vi "sorted data from csv.vi"(0 "cases CSV":string[][](array[string]), 2 "filter out":i32[](array[numeric]), 5 "US data":T1, 7 "Populations":i64[](array[numeric]), 9 "deaths CSV":string[][](array[string]), 11 "top selection":i32=5, 12 "SA data":T1, 13 "period in days to check":i32=7) -> (4 "ranked results":T2)   [LabVIEW 2019]
uses:
  <vilib>/Analysis/NI_AALPro.lvlib
panel:
  in  "last x days":i32=3
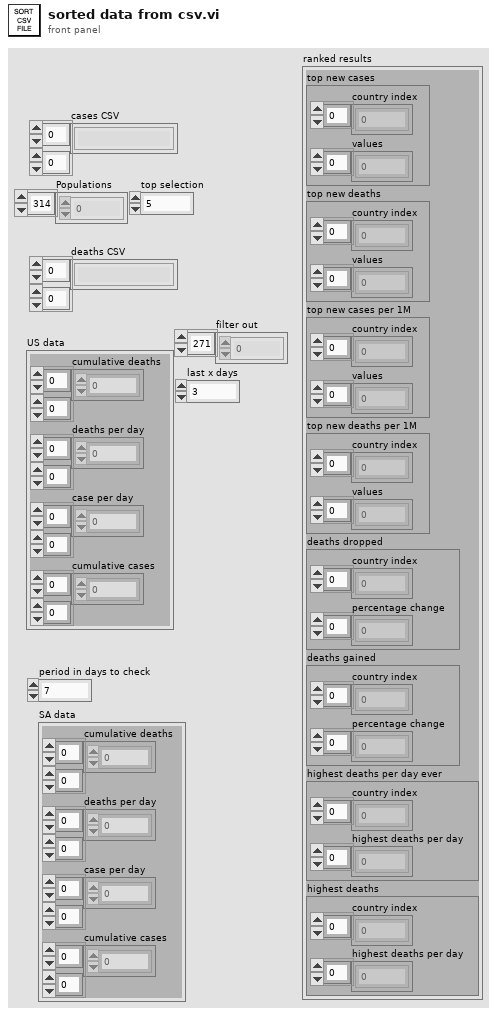
[diagram p1: front panel]
types:
  T1 = cluster{"cumulative deaths":i32[][], "deaths per day":i32[][], "case per day":i32[][], "cumulative cases":i32[][]}
  T2 = cluster{"top new cases":cluster{"country index":i32[], "values":i32[]}, "top new deaths":cluster{"country index":i32[], "values":i32[]}, "top new cases per 1M":cluster{"country index":i32[], "values":dbl[]}, "top new deaths per 1M":cluster{"country index":i32[], "values":dbl[]}, "deaths dropped":cluster{"country index":i32[], "percentage change":dbl[]}, "deaths gained":cluster{"country index":i32[], "percentage change":dbl[]}, "highest deaths per day ever":cluster{"country index":i32[], "highest deaths per day":dbl[]}, "highest deaths":cluster{"country index":i32[], "highest deaths per day":dbl[]}}
  T3 = cluster{"country index":i32[], "cumulative deaths per M":dbl[]}
  T4 = cluster{"country index":i32[], "highest deaths per day":dbl[]}
  T5 = cluster{"country index":i32[], "percentage change":dbl[]}
  T6 = cluster{"new deaths yesterday":dbl, "country index":i32}
  T7 = cluster{"new cases yesterday":dbl, "country index":i32}
  T8 = cluster{"percentage change":dbl, "country index":i32}
  T9 = cluster{"highest deaths per million":dbl, "country index":i32}
  T10 = cluster{"cumulative deaths per 1M":dbl, "country index":i32}
  T11 = cluster{"percentage change":dbl, "country index":i32}[]
  T12 = cluster{"new cases yesterday":dbl, "country index":i32}[]
  T13 = cluster{"new cases per 1M yesterday":dbl, "country index":i32}
  T14 = cluster{"new deaths yesterday":dbl, "country index":i32}[]
  T15 = cluster{"new deaths per 1M yesterday":dbl, "country index":i32}
  T16 = cluster{"new cases per 1M yesterday":dbl, "country index":i32}[]
  T17 = cluster{"new deaths per 1M yesterday":dbl, "country index":i32}[]
  T18 = cluster{"highest deaths per million":dbl, "country index":i32}[]
  T19 = cluster{"cumulative deaths per 1M":dbl, "country index":i32}[]
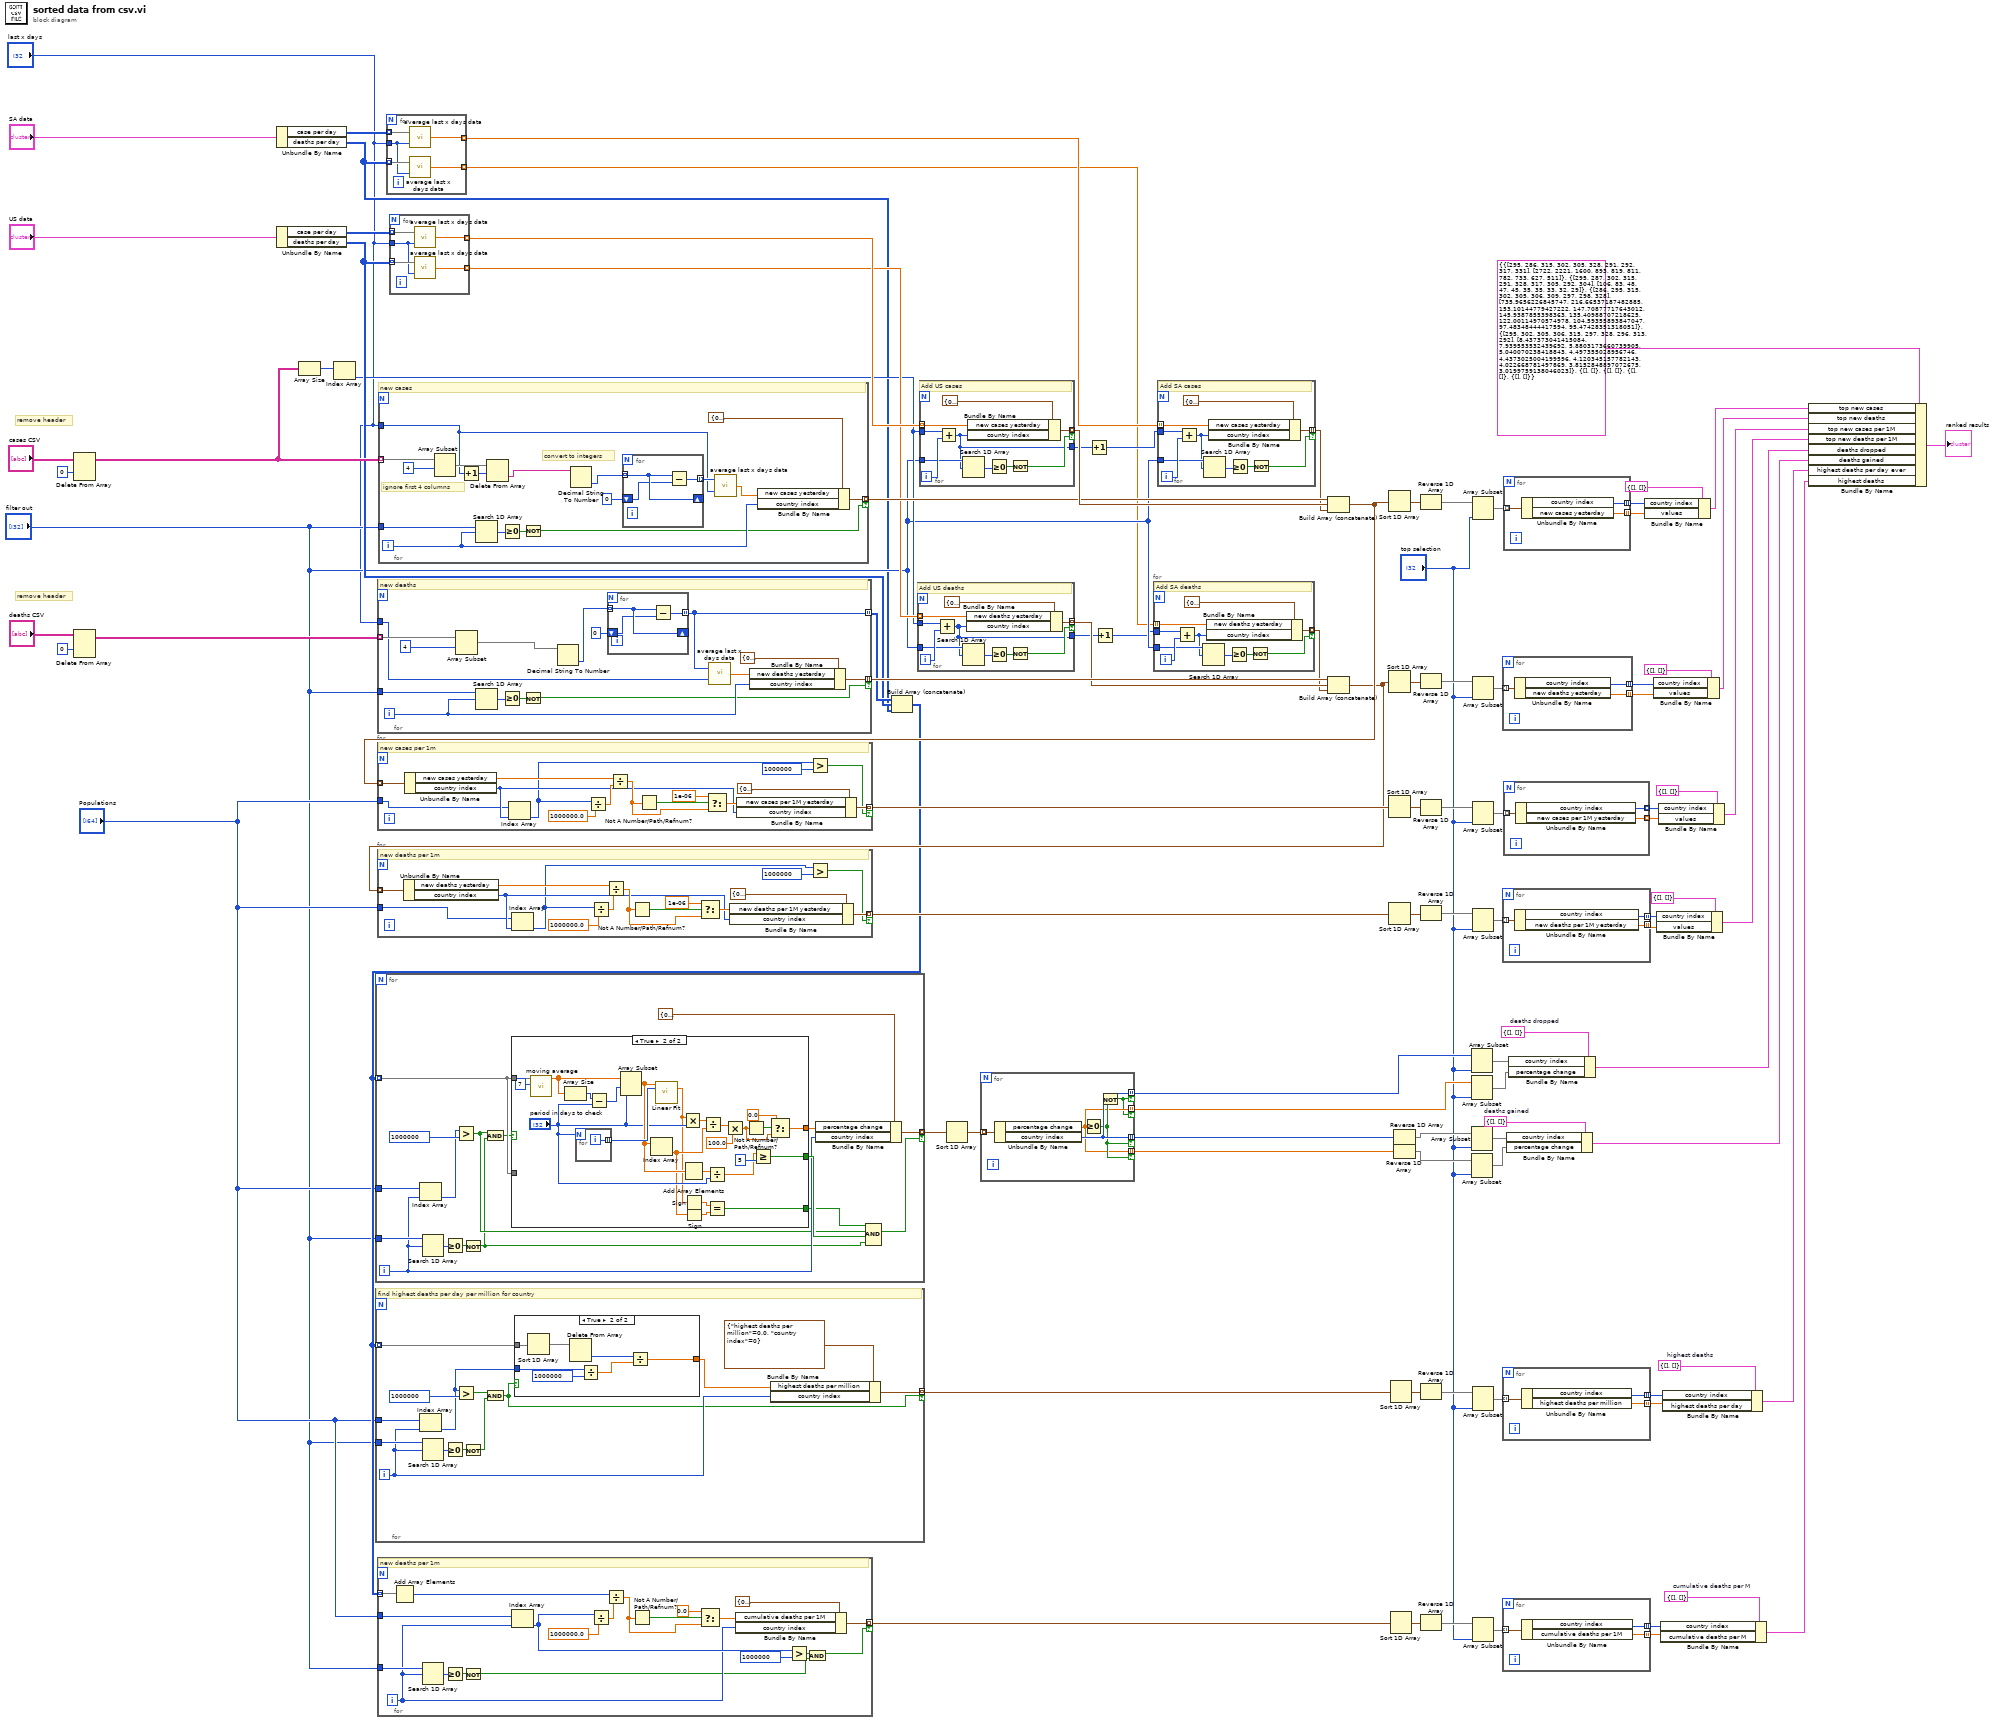
[diagram p0: block diagram]
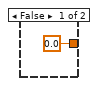
[diagram p2: hidden frame]
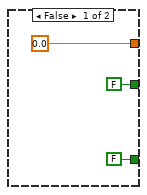
[diagram p3: hidden frame]
diagram:
  w21 = T3 {"country index"=[], "cumulative deaths per M"=[]}  # cumulative deaths per M
  w32 = T4 {"country index"=[], "highest deaths per day"=[]}  # highest deaths
  w47 = T5 {"country index"=[], "percentage change"=[]}  # deaths gained
  w48 = T5 {"country index"=[], "percentage change"=[]}  # deaths dropped
  # "remove header"
  # "remove header"
  n1 = Delete From Array(array="cases CSV", index (row)=0) -> (array with subset deleted=w72:string[][])  [unwired: 2 in, 1 out]
  n2 = Delete From Array(array="deaths CSV", index (row)=0) -> (array with subset deleted=w74:string[][])  [unwired: 2 in, 1 out]
  n3 = Unbundle By Name("SA data") -> ("case per day"=w14:i32[][], "deaths per day"=w2:i32[][])
  n4 = Unbundle By Name("US data") -> ("case per day"=w73:i32[][], "deaths per day"=w49:i32[][])
  n5 = Array Size(array=w72) -> (size(s)=w71:i32[])
  n6 = Index Array(array=w71) -> (element=w10:i32)  [unwired: 1 in]
  n7 = for {
    tunnel: w74 -> [w114] mode=indexing
    tunnel: [w112] -> w76 mode=indexing if=w106
    tunnel: "filter out" -> [w108]
    tunnel: [w101] -> w50 mode=indexing
    tunnel: "last x days" -> [w104]
    i -> [w107]
    # "new deaths"
    n8 = Array Subset(array=w114, index=4) -> (w111:string[])  [unwired: 1 in]
    n9 = Search 1D Array(1D array=w108, element=w107) -> (index of element=w109:i32)  [unwired: 1 in]
    n10 = Greater Or Equal To 0?(x=w109) -> (x >= 0?=w110:bool)
    n11 = Not(x=w110) -> (.not. x?=w106:bool)
    n12 = Decimal String To Number(string=w111) -> (number=w103:i32[])  [unwired: 2 in, 1 out]
    n13 = for {
      tunnel: w103 -> [w118] mode=indexing
      shift-right: [w118] -> _
      shift-left: 0 -> [w117]
      tunnel: [w116] -> w101 mode=indexing
      n14 = Subtract(x=w118, y=w117) -> (x-y=w116:i32)
    }
    n15 = call "average last x days data.vi"("last x days"=w104, "Array"=w101) -> ("avg last x days"=w102:dbl)
    n16 = Bundle By Name(cluster=T6 {"new deaths yesterday"=0.0, "country index"=0}, "new deaths yesterday"=w102, "country index"=w107) -> (w112:T6)
  }
  n17 = for {
    tunnel: w72 -> [w134] mode=indexing
    tunnel: [w132] -> w79 mode=indexing if=w127
    tunnel: "filter out" -> [w131]
    tunnel: "last x days" -> [w120]
    i -> [w130]
    # "convert to integers"
    # "ignore first 4 columns"
    # "new cases"
    n18 = Array Subset(array=w134, index=4) -> (w126:string[])  [unwired: 1 in]
    n19 = Increment(x=w120) -> (x+1=w125:i32)
    n20 = Search 1D Array(1D array=w131, element=w130) -> (index of element=w129:i32)  [unwired: 1 in]
    n21 = Delete From Array(array=w126, length=w125) -> (deleted portion=w124:string[])  [unwired: 1 in, 1 out]
    n22 = Greater Or Equal To 0?(x=w129) -> (x >= 0?=w128:bool)
    n23 = Not(x=w128) -> (.not. x?=w127:bool)
    n24 = Decimal String To Number(string=w124) -> (number=w122:i32[])  [unwired: 2 in, 1 out]
    n25 = for {
      tunnel: w122 -> [w138] mode=indexing
      shift-right: [w138] -> _
      shift-left: 0 -> [w137]
      tunnel: [w136] -> w121 mode=indexing
      n26 = Subtract(x=w138, y=w137) -> (x-y=w136:i32)
    }
    n27 = call "average last x days data.vi"("last x days"=w120, "Array"=w121) -> ("avg last x days"=w119:dbl)
    n28 = Bundle By Name(cluster=T7 {"new cases yesterday"=0.0, "country index"=0}, "new cases yesterday"=w119, "country index"=w130) -> (w132:T7)
  }
  n29 = for {
    tunnel: w14 -> [w142] mode=indexing
    tunnel: w2 -> [w143] mode=indexing
    tunnel: [w141] -> w11 mode=indexing
    tunnel: [w140] -> w3 mode=indexing
    tunnel: "last x days" -> [w139]
    n30 = call "average last x days data.vi"("last x days"=w139, "Array"=w142) -> ("avg last x days"=w141:dbl)
    n31 = call "average last x days data.vi"("last x days"=w139, "Array"=w143) -> ("avg last x days"=w140:dbl)
  }
  n32 = for {
    tunnel: w73 -> [w148] mode=indexing
    tunnel: w49 -> [w147] mode=indexing
    tunnel: [w145] -> w81 mode=indexing
    tunnel: [w146] -> w77 mode=indexing
    tunnel: "last x days" -> [w144]
    n33 = call "average last x days data.vi"("last x days"=w144, "Array"=w148) -> ("avg last x days"=w145:dbl)
    n34 = call "average last x days data.vi"("last x days"=w144, "Array"=w147) -> ("avg last x days"=w146:dbl)
  }
  n35 = Build Array (concatenate)(w50, w49, w2) -> (w26:i32[][])
  n36 = for {
    tunnel: w26 -> [w160] mode=indexing
    tunnel: "Populations" -> [w154]
    tunnel: [w162] -> w69 mode=indexing if=w161
    tunnel: "filter out" -> [w156]
    i -> [w155]
    n37 = Index Array(array=w154, index=w155) -> (element=w153:i64)
    n38 = Search 1D Array(1D array=w156, element=w155) -> (index of element=w157:i32)  [unwired: 1 in]
    n39 = Greater Or Equal To 0?(x=w157) -> (x >= 0?=w158:bool)
    n40 = Greater?(x=w153, y=1000000) -> (0:w151:bool)
    n41 = Not(x=w158) -> (.not. x?=w150:bool)
    n42 = And(x=w151, y=w150) -> (x .and. y?=w152:bool)
    n43 = case shown="True" w152 {
      tunnel: w160 -> [_ w192]
      tunnel: [0.0 w183] -> w163
      tunnel: [FALSE w181] -> w159
      tunnel: w160 -> [_ _]
      tunnel: [FALSE w169] -> w149
      frame False {
      }
      frame True {
        n44 = call "moving average.vi"("average over x points"=7, "Array"=w192) -> ("moving average array"=w191:dbl[])  [unwired: 8 in, 1 out]
        n45 = Array Size(array=w191) -> (size(s)=w190:i32)
        n46 = for {
          N: "period in days to check" -> [_]
          tunnel: [w193] -> w187 mode=indexing
          i -> [w193]
        }
        n47 = Subtract(x=w190, y="period in days to check") -> (x-y=w180:i32)
        n48 = Array Subset(array=w191, index=w180, length="period in days to check") -> (w177:dbl[])
        n49 = Index Array(array=w177) -> (element=w171:dbl)  [unwired: 1 in]
        n50 = call <vilib>:"Linear Fit.vi"("Y"=w177, "X"=w187) -> ("slope"=w170:dbl)  [unwired: 9 in, 4 out]
        n51 = Multiply(x=w170, y="period in days to check") -> (x*y=w189:dbl)
        n52 = Add Array Elements(numeric array=w177) -> (sum=w176:dbl)
        n53 = Sign(1:w170) -> (0:w172:dbl)
        n54 = Sign(1:w171) -> (0:w173:dbl)
        n55 = Divide(x=w189, y=w171) -> (x/y=w188:dbl)
        n56 = Divide(x=w176, y="period in days to check") -> (x/y=w174:dbl)
        n57 = Equal?(x=w172, y=w173) -> (x = y?=w169:bool)
        n58 = Multiply(x=w188, y=100.0) -> (x*y=w184:dbl)
        n59 = Not A Number/Path/Refnum?(number/path/refnum=w184) -> (NaN/Path/Refnum?=w186:bool)
        n60 = Greater Or Equal?(x=w174, y=5) -> (x >= y?=w181:bool)
        n61 = Select(t=0.0, s=w186, f=w184) -> (s? t:f=w183:dbl)
      }
    }
    n62 = Bundle By Name(cluster=T8 {"percentage change"=0.0, "country index"=0}, "percentage change"=w163, "country index"=w155) -> (w162:T8)
    n63 = Compound Arithmetic op=AND(w149, w151, w159, w150) -> (w161:bool)
  }
  n64 = for {
    tunnel: w26 -> [w197] mode=indexing
    tunnel: "Populations" -> [w200]
    tunnel: [w205] -> w35 mode=indexing if=w195
    tunnel: "filter out" -> [w202]
    i -> [w201]
    # "find highest deaths per day per million for country"
    n65 = Index Array(array=w200, index=w201) -> (element=w196:i64)
    n66 = Search 1D Array(1D array=w202, element=w201) -> (index of element=w203:i32)  [unwired: 1 in]
    n67 = Greater Or Equal To 0?(x=w203) -> (x >= 0?=w204:bool)
    n68 = Greater?(x=w196, y=1000000) -> (0:w199:bool)
    n69 = Not(x=w204) -> (.not. x?=w198:bool)
    n70 = And(x=w199, y=w198) -> (x .and. y?=w195:bool)
    n71 = case shown="True" w195 {
      tunnel: w197 -> [_ w215]
      tunnel: w196 -> [_ w214]
      tunnel: [0.0 w211] -> w194
      frame False {
      }
      frame True {
        n72 = Sort 1D Array(array=w215) -> (sorted array=w210:i32[])
        n73 = Delete From Array(array=w210) -> (deleted portion=w209:i32)  [unwired: 2 in, 1 out]
        n74 = Divide(x=w214, y=1000000) -> (x/y=w212:dbl)
        n75 = Divide(x=w209, y=w212) -> (x/y=w211:dbl)
      }
    }
    n76 = Bundle By Name(cluster=T9 {"highest deaths per million"=0.0, "country index"=0}, "highest deaths per million"=w194, "country index"=w201) -> (w205:T9)
  }
  n77 = for {
    tunnel: w26 -> [w223] mode=indexing
    tunnel: "Populations" -> [w225]
    tunnel: [w235] -> w18 mode=indexing if=w217
    tunnel: "filter out" -> [w219]
    i -> [w218]
    # "new deaths per 1m"
    n78 = Add Array Elements(numeric array=w223) -> (sum=w222:i32)
    n79 = Search 1D Array(1D array=w219, element=w218) -> (index of element=w221:i32)  [unwired: 1 in]
    n80 = Greater Or Equal To 0?(x=w221) -> (x >= 0?=w220:bool)
    n81 = Not(x=w220) -> (.not. x?=w216:bool)
    n82 = Index Array(array=w225, index=w218) -> (element=w224:i64)
    n83 = Divide(x=w224, y=1000000.0) -> (x/y=w232:dbl)
    n84 = Divide(x=w222, y=w232) -> (x/y=w230:dbl)
    n85 = Not A Number/Path/Refnum?(number/path/refnum=w230) -> (NaN/Path/Refnum?=w231:bool)
    n86 = Select(t=0.0, s=w231, f=w230) -> (s? t:f=w229:dbl)
    n87 = Bundle By Name(cluster=T10 {"cumulative deaths per 1M"=0.0, "country index"=0}, "cumulative deaths per 1M"=w229, "country index"=w218) -> (w235:T10)
    n88 = Greater?(x=w224, y=1000000) -> (0:w226:bool)
    n89 = And(x=w226, y=w216) -> (x .and. y?=w217:bool)
  }
  n90 = for {
    tunnel: w77 -> [w245] mode=indexing
    tunnel: w10 -> [w243]
    tunnel: [w242] -> w75 mode=indexing if=w238
    tunnel: "filter out" -> [w237]
    tunnel: [w236] -> w5
    i -> [w244]
    # "Add US deaths"
    n91 = Add(x=w243, y=w244) -> (x+y=w236:i32)
    n92 = Search 1D Array(1D array=w237, element=w236) -> (index of element=w239:i32)  [unwired: 1 in]
    n93 = Bundle By Name(cluster=T6 {"new deaths yesterday"=0.0, "country index"=0}, "new deaths yesterday"=w245, "country index"=w236) -> (w242:T6)
    n94 = Greater Or Equal To 0?(x=w239) -> (x >= 0?=w240:bool)
    n95 = Not(x=w240) -> (.not. x?=w238:bool)
  }
  n96 = for {
    tunnel: w81 -> [w254] mode=indexing
    tunnel: w10 -> [w253]
    tunnel: [w252] -> w80 mode=indexing if=w247
    tunnel: "filter out" -> [w248]
    tunnel: [w246] -> w9
    i -> [w249]
    # "Add US cases"
    n97 = Add(x=w253, y=w249) -> (x+y=w246:i32)
    n98 = Search 1D Array(1D array=w248, element=w246) -> (index of element=w251:i32)  [unwired: 1 in]
    n99 = Bundle By Name(cluster=T7 {"new cases yesterday"=0.0, "country index"=0}, "new cases yesterday"=w254, "country index"=w246) -> (w252:T7)
    n100 = Greater Or Equal To 0?(x=w251) -> (x >= 0?=w250:bool)
    n101 = Not(x=w250) -> (.not. x?=w247:bool)
  }
  n102 = Sort 1D Array(array=w69) -> (sorted array=w68:T11)
  n103 = for {
    tunnel: w68 -> [w260] mode=indexing
    tunnel: [w259] -> w70 mode=indexing if=w258
    tunnel: [w259] -> w43 mode=indexing if=w256
    tunnel: [w257] -> w46 mode=indexing if=w258
    tunnel: [w257] -> w41 mode=indexing if=w256
    n104 = Unbundle By Name(w260) -> ("percentage change"=w257:dbl, "country index"=w259:i32)
    n105 = Greater Or Equal To 0?(x=w257) -> (x >= 0?=w258:bool)
    n106 = Not(x=w258) -> (.not. x?=w256:bool)
  }
  n107 = Increment(x=w9) -> (x+1=w8:i32)
  n108 = Increment(x=w5) -> (x+1=w4:i32)
  n109 = for {
    tunnel: w3 -> [w270] mode=indexing
    tunnel: w4 -> [w268]
    tunnel: [w267] -> w7 mode=indexing if=w263
    tunnel: "filter out" -> [w262]
    i -> [w269]
    # "Add SA deaths"
    n110 = Add(x=w268, y=w269) -> (x+y=w261:i32)
    n111 = Search 1D Array(1D array=w262, element=w261) -> (index of element=w264:i32)  [unwired: 1 in]
    n112 = Bundle By Name(cluster=T6 {"new deaths yesterday"=0.0, "country index"=0}, "new deaths yesterday"=w270, "country index"=w261) -> (w267:T6)
    n113 = Greater Or Equal To 0?(x=w264) -> (x >= 0?=w265:bool)
    n114 = Not(x=w265) -> (.not. x?=w263:bool)
  }
  n115 = for {
    tunnel: w11 -> [w279] mode=indexing
    tunnel: w8 -> [w278]
    tunnel: [w277] -> w12 mode=indexing if=w272
    tunnel: "filter out" -> [w273]
    i -> [w274]
    # "Add SA cases"
    n116 = Add(x=w278, y=w274) -> (x+y=w271:i32)
    n117 = Search 1D Array(1D array=w273, element=w271) -> (index of element=w276:i32)  [unwired: 1 in]
    n118 = Bundle By Name(cluster=T7 {"new cases yesterday"=0.0, "country index"=0}, "new cases yesterday"=w279, "country index"=w271) -> (w277:T7)
    n119 = Greater Or Equal To 0?(x=w276) -> (x >= 0?=w275:bool)
    n120 = Not(x=w275) -> (.not. x?=w272:bool)
  }
  n121 = Build Array (concatenate)(w79, w80, w12) -> (w78:T12)
  n122 = for {
    tunnel: w78 -> [w295] mode=indexing
    tunnel: "Populations" -> [w282]
    tunnel: [w293] -> w84 mode=indexing if=w284
    # "new cases per 1m"
    n123 = Unbundle By Name(w295) -> ("new cases yesterday"=w291:dbl, "country index"=w283:i32)
    n124 = Index Array(array=w282, index=w283) -> (element=w281:i64)
    n125 = Divide(x=w281, y=1000000.0) -> (x/y=w290:dbl)
    n126 = Divide(x=w291, y=w290) -> (x/y=w287:dbl)
    n127 = Not A Number/Path/Refnum?(number/path/refnum=w287) -> (NaN/Path/Refnum?=w288:bool)
    n128 = Select(t=1e-06, s=w288, f=w287) -> (s? t:f=w286:dbl)
    n129 = Bundle By Name(cluster=T13 {"new cases per 1M yesterday"=0.0, "country index"=0}, "new cases per 1M yesterday"=w286, "country index"=w283) -> (w293:T13)
    n130 = Greater?(x=w281, y=1000000) -> (0:w284:bool)
  }
  n131 = Build Array (concatenate)(w76, w75, w7) -> (w27:T14)
  n132 = for {
    tunnel: w27 -> [w310] mode=indexing
    tunnel: "Populations" -> [w297]
    tunnel: [w309] -> w83 mode=indexing if=w299
    # "new deaths per 1m"
    n133 = Unbundle By Name(w310) -> ("new deaths yesterday"=w307:dbl, "country index"=w298:i32)
    n134 = Index Array(array=w297, index=w298) -> (element=w296:i64)
    n135 = Divide(x=w296, y=1000000.0) -> (x/y=w305:dbl)
    n136 = Divide(x=w307, y=w305) -> (x/y=w303:dbl)
    n137 = Not A Number/Path/Refnum?(number/path/refnum=w303) -> (NaN/Path/Refnum?=w304:bool)
    n138 = Select(t=1e-06, s=w304, f=w303) -> (s? t:f=w302:dbl)
    n139 = Bundle By Name(cluster=T15 {"new deaths per 1M yesterday"=0.0, "country index"=0}, "new deaths per 1M yesterday"=w302, "country index"=w298) -> (w309:T15)
    n140 = Greater?(x=w296, y=1000000) -> (0:w299:bool)
  }
  n141 = Sort 1D Array(array=w78) -> (sorted array=w96:T12)
  n142 = Sort 1D Array(array=w27) -> (sorted array=w95:T14)
  n143 = Sort 1D Array(array=w84) -> (sorted array=w85:T16)
  n144 = Sort 1D Array(array=w83) -> (sorted array=w86:T17)
  n145 = Sort 1D Array(array=w35) -> (sorted array=w33:T18)
  n146 = Sort 1D Array(array=w18) -> (sorted array=w20:T19)
  n147 = Reverse 1D Array(array=w70) -> (reversed array=w39:i32[])
  n148 = Reverse 1D Array(array=w46) -> (reversed array=w38:dbl[])
  n149 = Reverse 1D Array(array=w96) -> (reversed array=w94:T12)
  n150 = Reverse 1D Array(array=w95) -> (reversed array=w93:T14)
  n151 = Reverse 1D Array(array=w85) -> (reversed array=w87:T16)
  n152 = Reverse 1D Array(array=w86) -> (reversed array=w88:T17)
  n153 = Reverse 1D Array(array=w33) -> (reversed array=w34:T18)
  n154 = Reverse 1D Array(array=w20) -> (reversed array=w19:T19)
  n155 = Array Subset(array=w43, length="top selection") -> (w42:i32[])  [unwired: 1 in]
  n156 = Array Subset(array=w41, length="top selection") -> (w40:dbl[])  [unwired: 1 in]
  n157 = Array Subset(array=w39, length="top selection") -> (w37:i32[])  [unwired: 1 in]
  n158 = Array Subset(array=w38, length="top selection") -> (w36:dbl[])  [unwired: 1 in]
  n159 = Array Subset(array=w94, length="top selection") -> (w92:T12)  [unwired: 1 in]
  n160 = Array Subset(array=w93, length="top selection") -> (w91:T14)  [unwired: 1 in]
  n161 = Array Subset(array=w87, length="top selection") -> (w89:T16)  [unwired: 1 in]
  n162 = Array Subset(array=w88, length="top selection") -> (w90:T17)  [unwired: 1 in]
  n163 = Array Subset(array=w34, length="top selection") -> (w31:T18)  [unwired: 1 in]
  n164 = Array Subset(array=w19, length="top selection") -> (w22:T19)  [unwired: 1 in]
  n165 = for {
    tunnel: w91 -> [w313] mode=indexing
    tunnel: [w312] -> w61 mode=indexing
    tunnel: [w311] -> w60 mode=indexing
    n166 = Unbundle By Name(w313) -> ("country index"=w312:i32, "new deaths yesterday"=w311:dbl)
  }
  n167 = for {
    tunnel: w90 -> [w316] mode=indexing
    tunnel: [w315] -> w56 mode=indexing
    tunnel: [w314] -> w55 mode=indexing
    n168 = Unbundle By Name(w316) -> ("country index"=w315:i32, "new deaths per 1M yesterday"=w314:dbl)
  }
  n169 = for {
    tunnel: w31 -> [w319] mode=indexing
    tunnel: [w318] -> w30 mode=indexing
    tunnel: [w317] -> w29 mode=indexing
    n170 = Unbundle By Name(w319) -> ("country index"=w318:i32, "highest deaths per million"=w317:dbl)
  }
  n171 = for {
    tunnel: w22 -> [w322] mode=indexing
    tunnel: [w321] -> w23 mode=indexing
    tunnel: [w320] -> w24 mode=indexing
    n172 = Unbundle By Name(w322) -> ("country index"=w321:i32, "cumulative deaths per 1M"=w320:dbl)
  }
  n173 = for {
    tunnel: w92 -> [w325] mode=indexing
    tunnel: [w324] -> w65 mode=indexing
    tunnel: [w323] -> w64 mode=indexing
    n174 = Unbundle By Name(w325) -> ("country index"=w324:i32, "new cases yesterday"=w323:dbl)
  }
  n175 = for {
    tunnel: w89 -> [w328] mode=indexing
    tunnel: [w327] -> w54 mode=indexing
    tunnel: [w326] -> w53 mode=indexing
    n176 = Unbundle By Name(w328) -> ("country index"=w327:i32, "new cases per 1M yesterday"=w326:dbl)
  }
  n177 = Bundle By Name(cluster=w47, "country index"=w37, "percentage change"=w36) -> (w44:T5)
  n178 = Bundle By Name(cluster=w48, "country index"=w42, "percentage change"=w40) -> (w45:T5)
  n179 = Bundle By Name(cluster=cluster{"country index":i32[], "values":i32[]} {"country index"=[], "values"=[]} ("top new cases"), "country index"=w65, "values"=w64) -> (w63:cluster{"country index":i32[], "values":i32[]})
  n180 = Bundle By Name(cluster=cluster{"country index":i32[], "values":i32[]} {"country index"=[], "values"=[]} ("top new deaths"), "country index"=w61, "values"=w60) -> (w59:cluster{"country index":i32[], "values":i32[]})
  n181 = Bundle By Name(cluster=cluster{"country index":i32[], "values":dbl[]} {"country index"=[], "values"=[]} ("top new deaths per 1M"), "country index"=w56, "values"=w55) -> (w51:cluster{"country index":i32[], "values":dbl[]})
  n182 = Bundle By Name(cluster=cluster{"country index":i32[], "values":dbl[]} {"country index"=[], "values"=[]} ("top new cases per 1M"), "country index"=w54, "values"=w53) -> (w52:cluster{"country index":i32[], "values":dbl[]})
  n183 = Bundle By Name(cluster=w21, "country index"=w23, "cumulative deaths per M"=w24) -> (w16:T3)
  n184 = Bundle By Name(cluster=w32, "country index"=w30, "highest deaths per day"=w29) -> (w28:T4)
  n185 = Bundle By Name(cluster=T2 {"top new cases"={"country index"=[295, 286, 315, 302, 305, 328, 291, 292, 317, 331], "values"=[2722, 2221, 1600, 893, 819, 811, 782, 733, 627, 511]}, "top new deaths"={"country index"=[295, 287, 302, 315, 291, 328, 317, 305, 292, 304], "values"=[106, 83, 48, 47, 45, 35, 35, 33, 32, 29]}, "top new cases per 1M"={"country index"=[286, 295, 315, 302, 305, 306, 309, 297, 298, 328], "values"=[735.9656226845747, 216.66537187482885, 153.10144779427222, 147.70877717643012, 145.9387855398363, 135.40988707218625, 122.00114970574978, 104.59355893847047, 97.48348444417594, 95.47428351318051]}, "top new deaths per 1M"={"country index"=[295, 302, 305, 306, 315, 297, 328, 296, 313, 292], "values"=[8.437373041415084, 7.939553532439692, 5.8803173660739905, 5.040070238418843, 4.497355028956746, 4.4373025004199596, 4.120345157782143, 4.022668781497869, 3.8152848897072675, 3.0199759138046023]}, "deaths dropped"={"country index"=[], "percentage change"=[]}, "deaths gained"={"country index"=[], "percentage change"=[]}, "highest deaths per day ever"={"country index"=[], "highest deaths per day"=[]}, "highest deaths"={"country index"=[], "highest deaths per day"=[]}}, "top new cases"=w63, "top new deaths"=w59, "top new cases per 1M"=w52, "top new deaths per 1M"=w51, "deaths dropped"=w45, "deaths gained"=w44, "highest deaths per day ever"=w28, "highest deaths"=w16) -> (→"ranked results":T2)
